vi "Security System Demo Machine Based.vi"() -> ()   [LabVIEW 2016]
doc: "This Main VI of Security System Software Demo project is developed based on State Machine design pattern."
uses:
  Controls/States.ctl
  Controls/Module Data.ctl
  Controls/Zone Status Indicators.ctl
panel:
  in  "error In":errorcluster
  in  "Alarm Switches":bool[](array[boolean])=[FALSE, FALSE, FALSE, FALSE, FALSE, FALSE, FALSE]
  in  "Bypass Switches":bool[](array[boolean])=[FALSE, FALSE, FALSE, FALSE, FALSE, FALSE, FALSE]
  in  "Tamper Switches":bool[](array[boolean])=[FALSE, FALSE, FALSE, FALSE, FALSE, FALSE]
  out "Zone Status Indicators":T1 caption="Green    = Normal\nRed       =  Alarm\nOrange = Tamper\nBlue      = Bypass"
  in  "Stop":bool
  # "1"
  # "2"
  # "3"
  # "4"
  # "5"
  # "6"
  # "Zone"
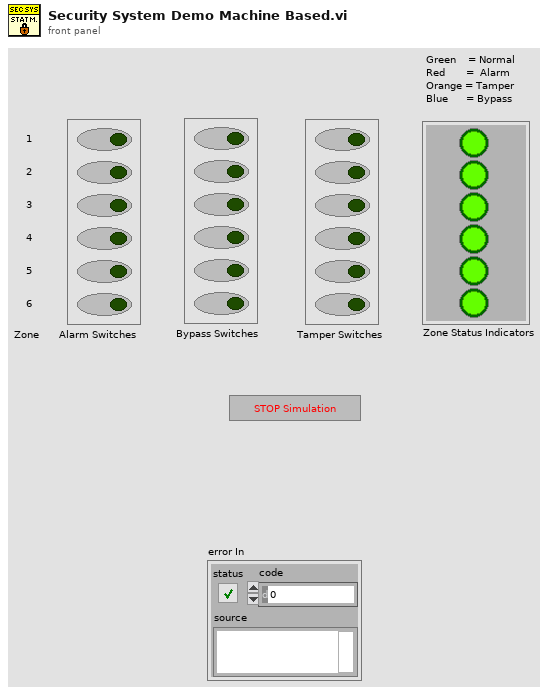
[diagram p1: front panel]
types:
  T1 = typedef "Zone Status Indicators.ctl" = cluster{"Boolean":bool, "Boolean 2":bool, "Boolean 3":bool, "Boolean 4":bool, "Boolean 5":bool, "Boolean 6":bool}
  T2 = typedef "Module Data.ctl" = cluster{"Controls[]":refnum<vi>[], "Zone Status Data":string[]}
  T3 = typedef "States.ctl" = enum16{"Initialize", "Get Event", "Log to File", "Exit"}
  T4 = typedef "Zones Condition.ctl" = enum16{"Normal", "Bypass", "Tamper", "Alarm"}
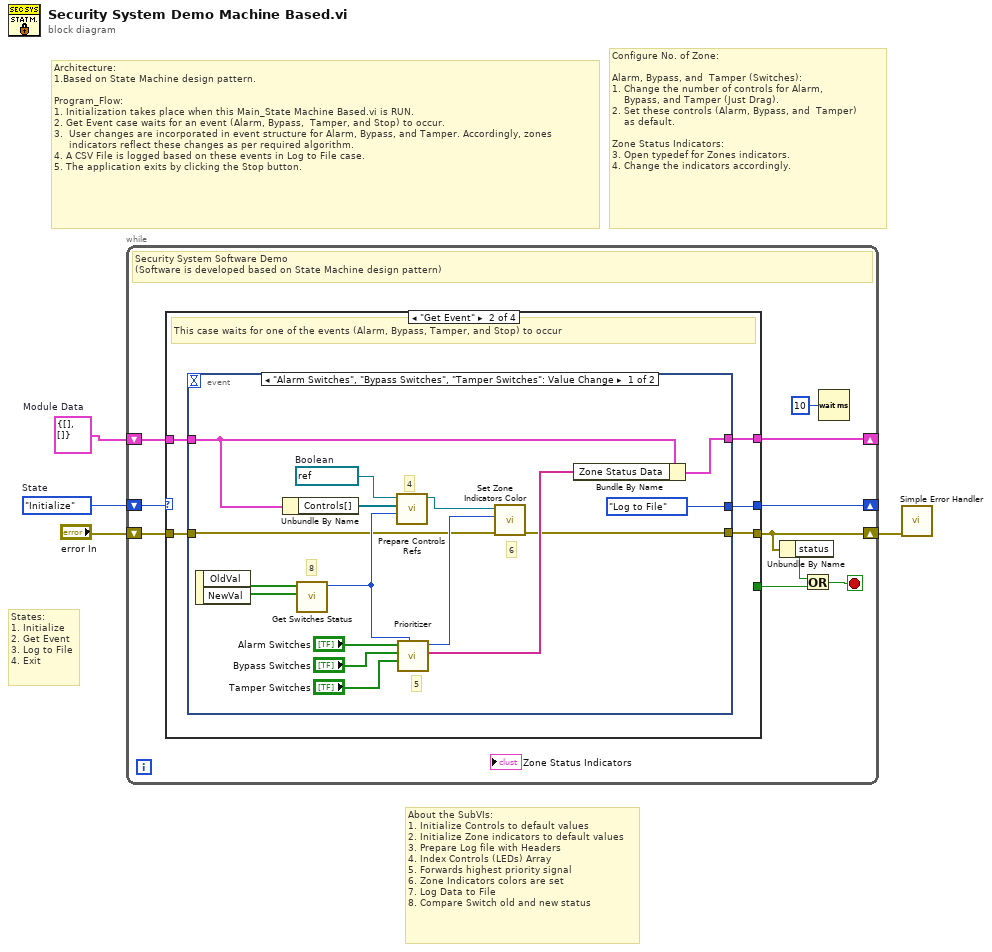
[diagram p0: block diagram]
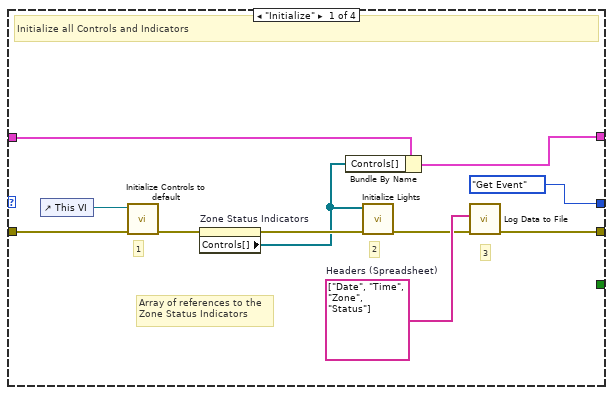
[diagram p2: hidden frame]
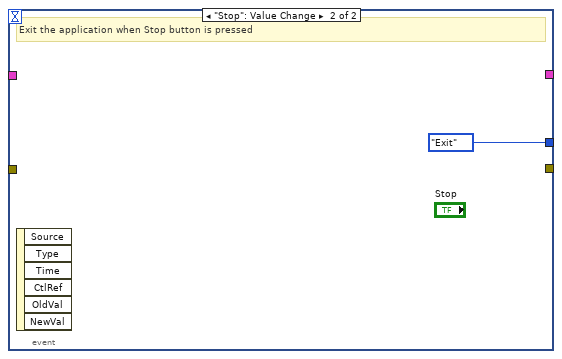
[diagram p3: hidden frame]
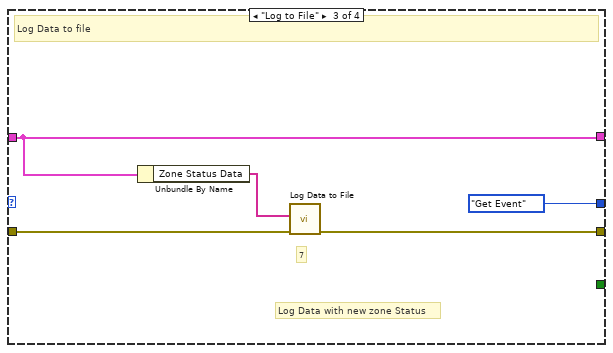
[diagram p4: hidden frame]
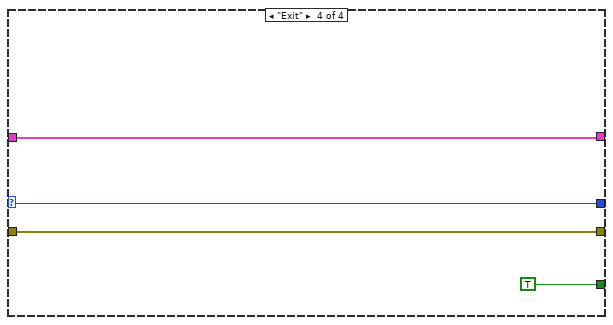
[diagram p5: hidden frame]
diagram:
  w2 = T2 {"Controls[]"=[], "Zone Status Data"=[]}  # Module Data
  w3 = States."Initialize"  # State
  # "States:\n1. Initialize\n2. Get Event\n3. Log to File\n4. Exit"
  # "Configure No. of Zone:\n\nAlarm, Bypass, and  Tamper (Switches):\n1. Change the number of controls for Alarm, \n    Bypass, and Tamper (Just Drag).\n2. Set these controls (Alarm, Bypass, and  Tamper) \n    as default.\n\nZone Status Indicators:\n3. Open typedef for Zones indicators.\n4. Change the indicators accordingly."
  # "Architecture:\n1.Based on State Machine design pattern.  \n\nProgram_Flow:\n1. Initialization takes place when this Main_State Machine Based.vi is RUN.\n2. Get Event case waits for an event (Alarm, Bypass,  Tamper, and Stop) to occur.\n3.  User changes are incorporated in event structure for Alarm, Bypass, and Tamper. Accordingly, zones \n     indicators reflect these changes as per required algorithm.\n4. A CSV File is logged based on these events in Log to File case.\n5. The application exits by clicking the Stop button."
  # "About the SubVIs:\n1. Initialize Controls to default values\n2. Initialize Zone indicators to default values\n3. Prepare Log file with Headers\n4. Index Controls (LEDs) Array \n5. Forwards highest priority signal\n6. Zone Indicators colors are set\n7. Log Data to File\n8. Compare Switch old and new status"
  n1 = while {
    shift-right: [w13] -> _
    shift-left: w3 -> [w6]
    shift-right: [w12] -> w4
    shift-left: "error In" -> [w14]
    shift-right: [w8] -> _
    shift-left: w2 -> [w7]
    stop <- w9 stop-if-true
    # "Security System Software Demo\n(Software is developed based on State Machine design pattern)"
    n2 = case shown="\"Get Event\"" w6 {
      selector: w6 -> [_ _ _ w53]
      tunnel: w14 -> [w24 w28 w50 w54]
      tunnel: [w22 w27 w49 w54] -> w12
      tunnel: [States."Get Event" ("Commands") w26 States."Get Event" ("Commands") w53] -> w13
      tunnel: [_ _ _ TRUE] -> w10
      tunnel: w7 -> [w20 w30 w52 w55]
      tunnel: [w18 w29 w52 w55] -> w8
      frame "Initialize" {
        w23 = string[] ["Date", "Time", "Zone", "Status"]  # Headers (Spreadsheet)
        # "3"
        # "2"
        # "1"
        # "Array of references to the\nZone Status Indicators"
        # "Initialize all Controls and Indicators"
        n3 = control-ref of="This VI"() -> (w25:refnum<vi>)
        n4 = call "Initialize Controls to default.vi"("error in (no error)"=w24, "VI in"=w25) -> ("error out"=w16:errorcluster)  [unwired: 9 in]
        n5 = property on="Zone Status Indicators" class="Clust (strict)"(error in=w16) -> (error out=w21:errorcluster, "Controls[]"=w19:refnum<vi>[])  [unwired: 1 in, 1 out]
        n6 = Bundle By Name(cluster=w20, "Controls[]"=w19) -> (w18:T2)
        n7 = call "Initialize Lights.vi"("error in (no error)"=w21, "Controls[]"=w19) -> ("error out"=w17:errorcluster)  [unwired: 9 in]
        n8 = call "Log Data to File.vi"("error in"=w17, "Log Data"=w23) -> ("error out"=w22:errorcluster)  [unwired: 9 in]
      }
      frame "Get Event" {
        # "This case waits for one of the events (Alarm, Bypass, Tamper, and Stop) to occur"
        n9 = event shown="[0] \"Alarm Switches\", \"Bypass Switches\", \"Tamper Switches\": Value Change" {
          selector: _ -> [_ _]
          dyn-events: _ -> [_ _]
          timeout: _ -> [_ _]
          tunnel: w30 -> [w37 _]
          tunnel: [w36 _] -> w29
          tunnel: w28 -> [w33 _]
          tunnel: [w32 _] -> w27
          tunnel: [States."Log to File" ("Commands") States."Exit" ("Commands")] -> w26
          event "Alarm Switches", "Bypass Switches", "Tamper Switches": Value Change {
            w38 = refnum<vi> refnum  # Boolean
            # "6"
            # "5"
            # "4"
            # "8"
            n10 = event-data() -> ("OldVal"=w35:bool[], "NewVal"=w34:bool[])  [unwired: 1 in]
            n11 = Unbundle By Name(w37) -> ("Controls[]"=w40:refnum<vi>[])
            n12 = call "Get Switches Status.vi"("NewVal"=w34, "OldVal"=w35) -> ("Zone Number - 1"=w41:i32)  [unwired: 9 in]
            n13 = call "Prepare Controls Refs.vi"("Numeric"=w41, "Controls[]"=w40, "Boolean in"=w38) -> ("Boolean out"=w42:refnum<vi>)  [unwired: 8 in]
            n14 = call "Prioritizer.vi"("Zone"=w41, "Tamper Switches"="Tamper Switches", "Bypass Switches"="Bypass Switches", "Alarm Switches"="Alarm Switches") -> ("Zone Status Data"=w39:string[], "Zone Condition"=w43:T4)  [unwired: 6 in]
            n15 = call "Set Zone Indicators Color.vi"("error in"=w33, "Alert Status"=w43, "reference"=w42) -> ("error out"=w32:errorcluster)  [unwired: 8 in]
            n16 = Bundle By Name(cluster=w37, "Zone Status Data"=w39) -> (w36:T2)
          }
          event "Stop": Value Change {
            # "Exit the application when Stop button is pressed"
            n17 = event-data() -> ()  [unwired: 1 in, 6 out]
          }
        }
      }
      frame "Log to File" {
        # "7"
        # "Log Data with new zone Status"
        # "Log Data to file"
        n18 = Unbundle By Name(w52) -> ("Zone Status Data"=w51:string[])
        n19 = call "Log Data to File.vi"("error in"=w50, "Log Data"=w51) -> ("error out"=w49:errorcluster)  [unwired: 9 in]
      }
      frame "Exit" {
      }
    }
    n20 = Unbundle By Name(w12) -> ("status"=w11:bool)
    n21 = Or(x=w11, y=w10) -> (x .or. y?=w9:bool)
    n22 = Wait (ms)(milliseconds to wait=u32 10) -> ()  [unwired: 1 out]
  }
  n23 = call <vilib>:"Simple Error Handler.vi"("error in (no error)"=w4) -> ()  [unwired: 4 in, 5 out]
